vi "Measurement Logic.vi"(8 "error in":errorcluster, 9 "measurement configuration":T3={"double array in"=[3.4, 5.6], "double in"=1.2, "U32 array in"=[32, 33], "U32 in"=32, "U64 array in"=[64, 65], "U64 in"=64, "I32 array in"=[-32, -33], "I32 in"=-32, "I64 array in"=[-64, -65], "I64 in"=-64, "bool in"=TRUE, "string in"="Lorem ipsum dolor sit", "u32 color ring in"=1, "u32 animal enum in"=enum."Gopher"} {"u32 color ring in" items=["Red", "Green", "Blue"]}, 10 "measure call context in":refnum<class "Measure Call Context.lvclass">, 11 "Stop OOB Server UE":refnum<user-event>) -> (0 "error out":errorcluster, 1 "measurement results":T1={"xy data out"={"x_data"=[], "y_data"=[]}, "double array out"=[0.0], "double out"=0.0, "U32 array out"=[0], "U32 out"=0, "U64 array out"=[0], "U64 out"=0, "I32 array out"=[0], "I32 out"=0, "I64 array out"=[0], "I64 out"=0, "bool out"=FALSE, "u32 color ring out"=0, "u32 animal enum out"=enum."Rabbit", "OOB Port"=0, "PauseResume out"=FALSE, "Export out"="", "string out"="Empty"} {"u32 color ring out" items=["Red", "Green", "Blue"]}, 2 "measure call context out":refnum<class "Measure Call Context.lvclass">)   [LabVIEW 2025, in "Example Plugin.lvclass"]
doc: "Contains the core logic for executing the measurement."
uses:
  Example Plugin.lvclass
  <vilib>/Plug-In SDKs/Measurements/Measure Call Context/Measure Call Context.lvclass
  Measurement Configuration.ctl
  Measurement Results.ctl
  <vilib>/gRPC/Generated APIs/ni/protobuf/types/RPC Messages/ni_protobuf_types_DoubleXYData.ctl
  <vilib>/gRPC/Generated APIs/ni/protobuf/types/ni.protobuf.types.lvlib
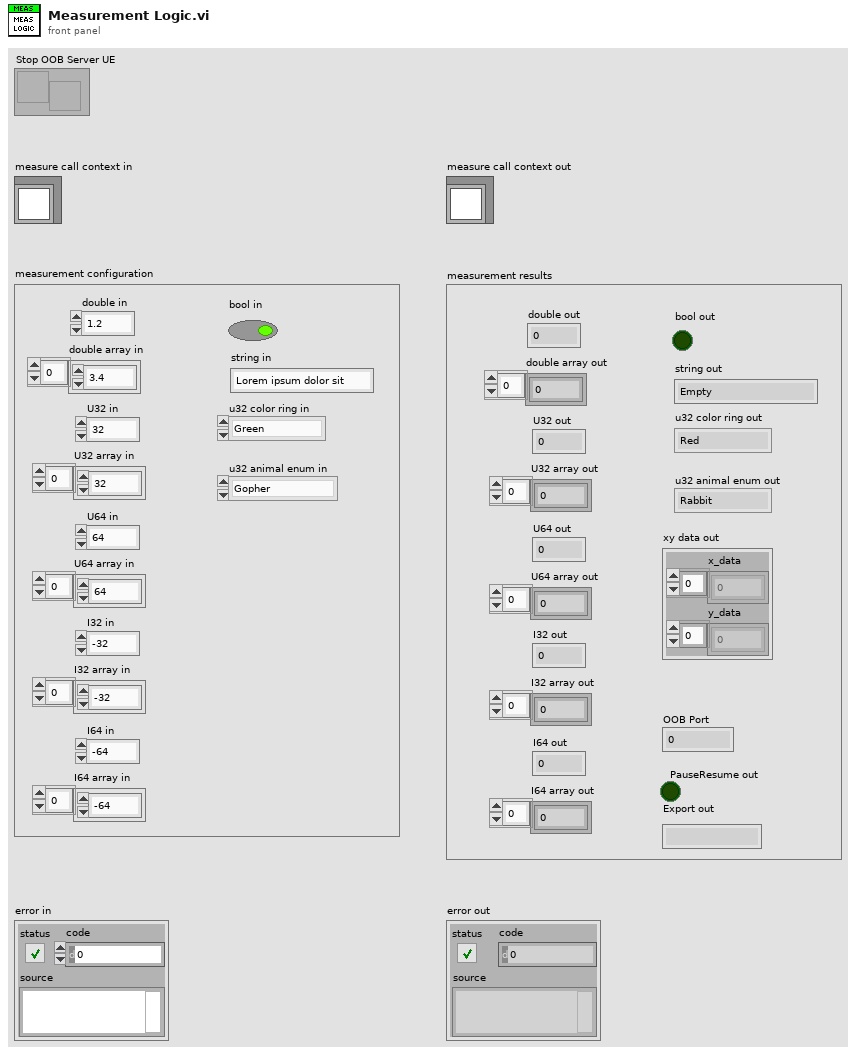
[diagram p1: front panel]
types:
  T1 = typedef "Example Plugin.lvclass/Measurement Results.ctl" = cluster{"xy data out":T2, "double array out":dbl[], "double out":dbl, "U32 array out":u32[], "U32 out":u32, "U64 array out":u64[], "U64 out":u64, "I32 array out":i32[], "I32 out":i32, "I64 array out":i64[], "I64 out":i64, "bool out":bool, "u32 color ring out":u32, "u32 animal enum out":enum32{"Rabbit", "Gopher", "Badger"}, "OOB Port":i32, "PauseResume out":bool, "Export out":string, "string out":string}
  T2 = typedef "ni.protobuf.types.lvlib/ni_protobuf_types_DoubleXYData.ctl" = cluster{"x_data":dbl[], "y_data":dbl[]}
  T3 = typedef "Example Plugin.lvclass/Measurement Configuration.ctl" = cluster{"double array in":dbl[], "double in":dbl, "U32 array in":u32[], "U32 in":u32, "U64 array in":u64[], "U64 in":u64, "I32 array in":i32[], "I32 in":i32, "I64 array in":i64[], "I64 in":i64, "bool in":bool, "string in":string, "u32 color ring in":u32, "u32 animal enum in":enum32{"Rabbit", "Gopher", "Badger"}}
  T4 = typedef "Example Plugin.lvclass/OOB to Logic Data.ctl" = cluster{"PauseResume":bool, "Export":string}
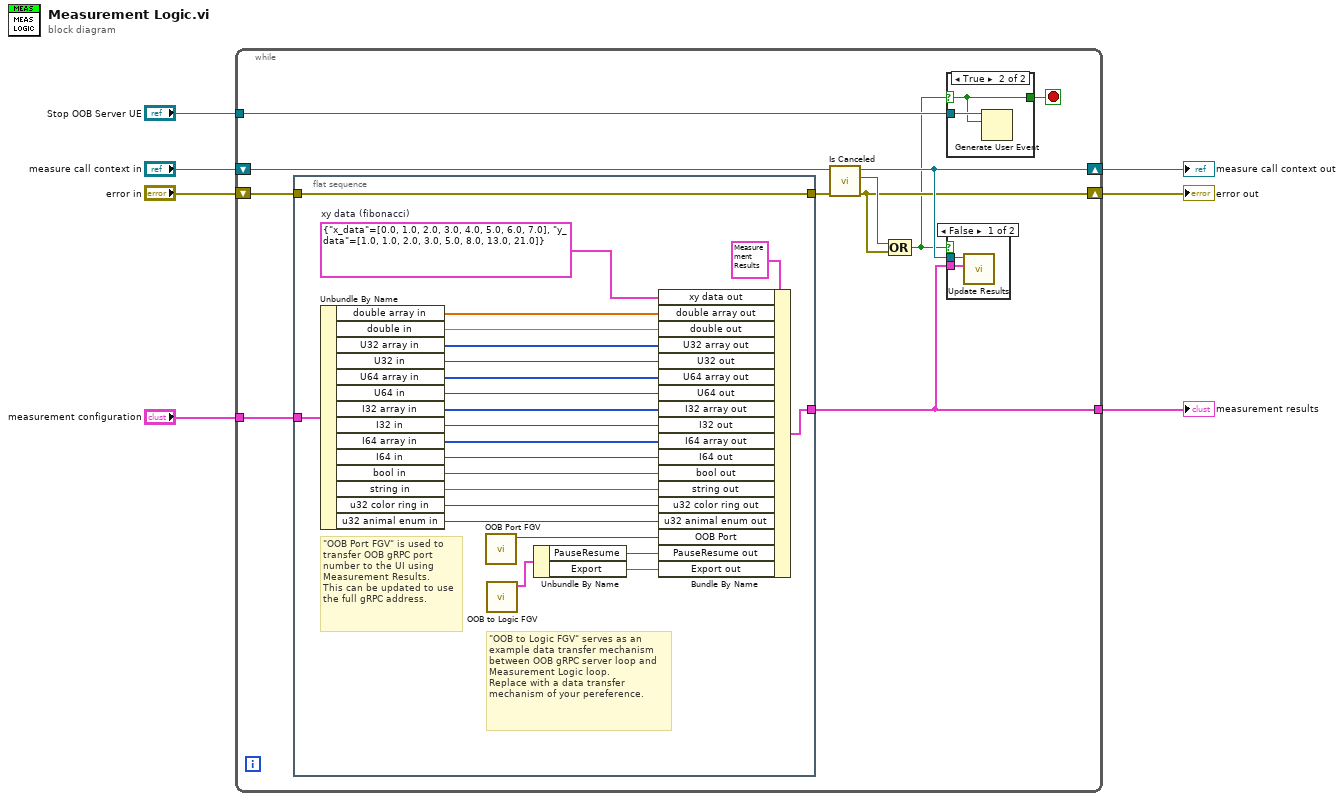
[diagram p0: block diagram]
diagram:
  n1 = while {
    tunnel: "measurement configuration" -> [w18]
    tunnel: [w15] -> w6
    shift-right: [w13] -> w2
    shift-left: "measure call context in" -> [w16]
    shift-right: [w10] -> w4
    shift-left: "error in" -> [w17]
    tunnel: "Stop OOB Server UE" -> [w12]
    stop <- w8 stop-if-true
    n2 = flat-sequence {
      tunnel: w18 -> [w30]
      tunnel: [w29] -> w15
      tunnel: w17 -> [w28]
      tunnel: [w28] -> w14
      frame #0 {
        w31 = T2 {"x_data"=[0.0, 1.0, 2.0, 3.0, 4.0, 5.0, 6.0, 7.0], "y_data"=[1.0, 1.0, 2.0, 3.0, 5.0, 8.0, 13.0, 21.0]}  # xy data (fibonacci)
        # "\"OOB Port FGV\" is used to transfer OOB gRPC port number to the UI using Measurement Results.\nThis can be updated to use the full gRPC address."
        # "\"OOB to Logic FGV\" serves as an example data transfer mechanism between OOB gRPC server loop and Measurement Logic loop.\nReplace with a data transfer mechanism of your pereference."
        n3 = Unbundle By Name(w30) -> ("double array in"=w45:dbl[], "double in"=w44:dbl, "U32 array in"=w43:u32[], "U32 in"=w42:u32, "U64 array in"=w41:u64[], "U64 in"=w40:u64, "I32 array in"=w39:i32[], "I32 in"=w38:i32, "I64 array in"=w37:i64[], "I64 in"=w36:i64, "bool in"=w35:bool, "string in"=w34:string, "u32 color ring in"=w33:u32, "u32 animal enum in"=w32:enum32{"Rabbit", "Gopher", "Badger"})
        n4 = call "OOB Port FGV.vi"() -> ("Listening Port out"=w27:i32)  [unwired: 11 in]
        n5 = call "OOB to Logic FGV.vi"() -> ("OOB to Logic Data out"=w26:T4)  [unwired: 10 in, 1 out]
        n6 = Unbundle By Name(w26) -> ("PauseResume"=w25:bool, "Export"=w24:string)
        n7 = Bundle By Name(cluster=T1 {"xy data out"={"x_data"=[], "y_data"=[]}, "double array out"=[], "double out"=0.0, "U32 array out"=[0], "U32 out"=0, "U64 array out"=[0], "U64 out"=0, "I32 array out"=[0], "I32 out"=0, "I64 array out"=[0], "I64 out"=0, "bool out"=FALSE, "u32 color ring out"=0, "u32 animal enum out"=enum."Rabbit", "OOB Port"=0, "PauseResume out"=FALSE, "Export out"="", "string out"="Empty"} ("Measurement Results"), "xy data out"=w31, "double array out"=w45, "double out"=w44, "U32 array out"=w43, "U32 out"=w42, "U64 array out"=w41, "U64 out"=w40, "I32 array out"=w39, "I32 out"=w38, "I64 array out"=w37, "I64 out"=w36, "bool out"=w35, "string out"=w34, "u32 color ring out"=w33, "u32 animal enum out"=w32, "OOB Port"=w27, "PauseResume out"=w25, "Export out"=w24) -> (w29:T1)
      }
    }
    n8 = call <vilib>:"Is Canceled.vi"("error in"=w14, "measure call context in"=w16) -> ("error out"=w10:errorcluster, "is canceled?"=w11:bool, "measure call context out"=w13:refnum<class "Measure Call Context.lvclass">)  [unwired: 7 in]
    n9 = Compound Arithmetic op=OR(w11, w10) -> (w9:bool)
    n10 = case shown="True" w9 {
      selector: w9 -> [w19 w20]
      tunnel: w12 -> [_ w21]
      tunnel: [w19 w20] -> w8
      frame False {
      }
      frame True {
        n11 = Generate User Event(user event=w21, event data cluster=w20) -> ()  [unwired: 2 in, 2 out]
      }
    }
    n12 = case shown="False" w9 {
      tunnel: w13 -> [w23 _]
      tunnel: w15 -> [w22 _]
      frame False {
        n13 = call <vilib>:"Update Results.vi"("measurement results"=w22, "measure call context in"=w23) -> ()  [unwired: 8 in, 2 out]
      }
      frame True {
      }
    }
  }
  "error out" <- w4
  "measure call context out" <- w2
  "measurement results" <- w6
